vi "Rd Wr settings json Filter Wheel Table.vi"(8 "error in (no error)":errorcluster, 9 "Settings File":string="FilterWheelTable.json", 10 "Write? (F:Read)":bool, 11 "Filter Wheel Table":cluster{i32[], bool}[][](array[cluster])=[[{[], TRUE}, {[2800], TRUE}, {[2800, 2800], TRUE}, {[950, 1850], FALSE}], [{[2800], FALSE}, {[], TRUE}, {[2800], TRUE}, {[2800, 2800], TRUE}], [{[2800, 2800], FALSE}, {[2800], FALSE}, {[], TRUE}, {[2800], TRUE}], [{[2800, 2800], TRUE}, {[2800, 2800], FALSE}, {[2800], FALSE}, {[], TRUE}]]) -> (0 "error out":errorcluster, 3 "Filter Wheel Table":cluster{i32[], bool}[][](array[cluster])=[[{[], TRUE}, {[2800], TRUE}, {[2800, 2800], TRUE}, {[950, 1850], FALSE}], [{[2800], FALSE}, {[], TRUE}, {[2800], TRUE}, {[2800, 2800], TRUE}], [{[2800, 2800], FALSE}, {[2800], FALSE}, {[], TRUE}, {[2800], TRUE}], [{[2800, 2800], TRUE}, {[2800, 2800], FALSE}, {[2800], FALSE}, {[], TRUE}]])   [LabVIEW 2024]
uses:
  2e80df6d-94aa-46b9-8b94-ceea8c057880.vi
  659fb017-0e9f-42f9-b06e-930303f00cbc.vi
  <vilib>/JDP Science/JSONtext/Find Item.vi
  <vilib>/JDP Science/JSONtext/Next JSON Value.vi
  <vilib>/JDP Science/JSONtext/String Subset.vi
  <vilib>/JDP Science/JSONtext/Parsing/Advance past next JSON Value (inlined COPY).vi
  <vilib>/JDP Science/JSONtext/Parsing/Advance past whitespace.vi
  <vilib>/JDP Science/JSONtext/Parsing/Advance past String.vi
  <vilib>/JDP Science/JSONtext/Parsing/Advance past Number.vi
  <vilib>/JDP Science/JSONtext/Parsing/Advance past Line Ending.vi
  <vilib>/JDP Science/JSONtext/Parsing/Parse Full Path or Item Name.vi
  <vilib>/JDP Science/JSONtext/Parsing/Advance past Array.vi
  <vilib>/JDP Science/JSONtext/Parsing/Advance past Object.vi
  <vilib>/JDP Science/JSONtext/support/Error Cluster From Code.vi
  <vilib>/JDP Science/JSONtext/Offset/Find Item Locations by Path.vi
  <vilib>/JDP Science/JSONtext/JSON text to Variant.vi
  <vilib>/JDP Science/JSONtext/Variant to JSON Text.vi
  <vilib>/JDP Science/JSONtext/Set Item.vi
  <vilib>/JDP Science/JSONtext/LVClass Serializer/JSONtext LVClass Serializer.lvclass
  <vilib>/JDP Science/JSONtext/JSONtext.lvlib
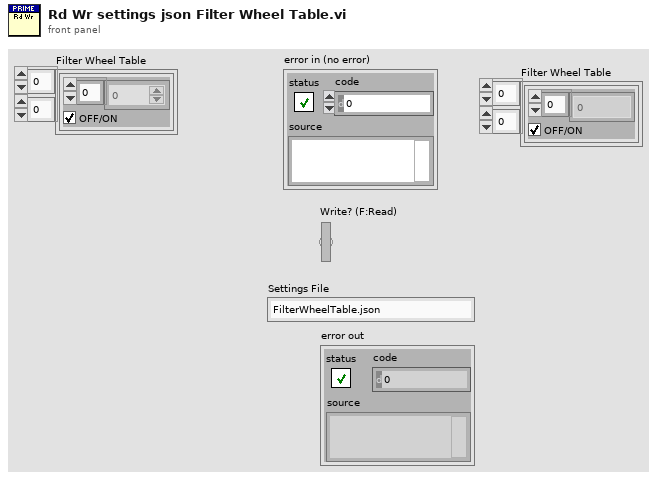
[diagram p1: front panel]
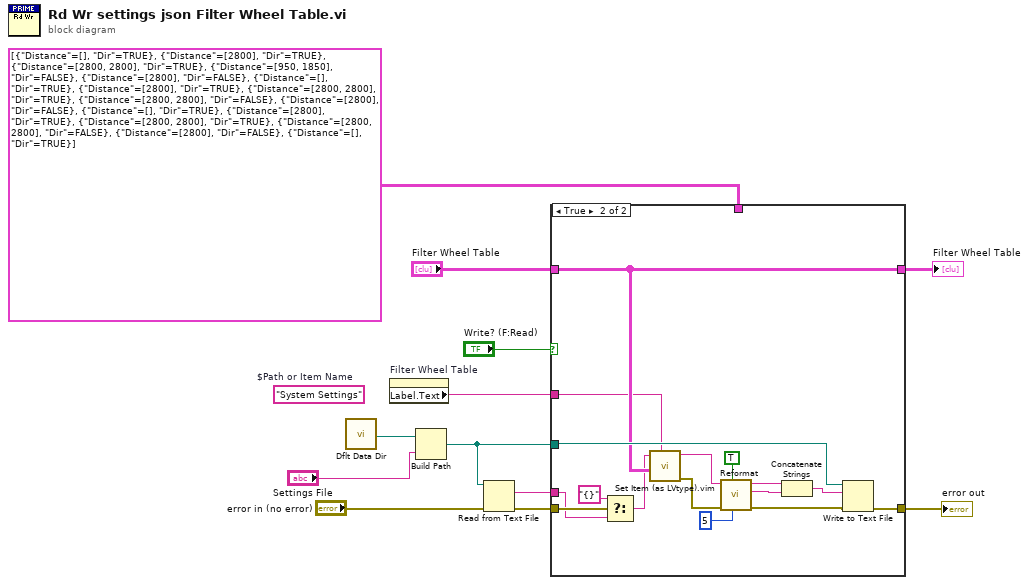
[diagram p0: block diagram]
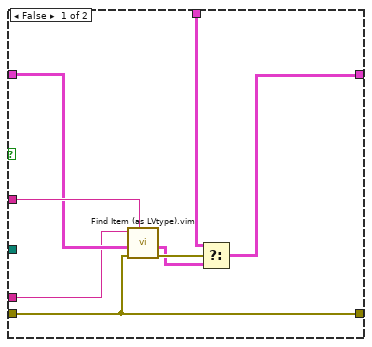
[diagram p2: hidden frame]
diagram:
  (unwired) "System Settings"  # $Path or Item Name
  n1 = call <vilib>:"Dflt Data Dir.vi"() -> ("App:Default Data Directory"=w9:path)
  n2 = property on="Filter Wheel Table" class="Arr (strict)"() -> ("Label.Text"=w2:string)  [unwired: 2 in, 2 out]
  n3 = Build Path(base path=w9, name or relative path="Settings File") -> (appended path=w3:path)
  n4 = Read from Text File(file (use dialog)=w3, error in="error in (no error)") -> (text=w4:string, error out=w5:errorcluster)  [unwired: 2 in, 2 out]
  n5 = case shown="True" "Write? (F:Read)" {
    tunnel: w5 -> [w14 w32]
    tunnel: "Filter Wheel Table" -> [w18 w34]
    tunnel: w3 -> [_ w36]
    tunnel: [w14 w35] -> w8
    tunnel: [w20 w34] -> w7
    tunnel: w2 -> [w19 w33]
    tunnel: w4 -> [w15 w30]
    tunnel: cluster{"Distance":i32[], "Dir":bool}[][] [[{"Distance"=[], "Dir"=TRUE}, {"Distance"=[2800], "Dir"=TRUE}, {"Distance"=[2800, 2800], "Dir"=TRUE}, {"Distance"=[950, 1850], "Dir"=FALSE}], [{"Distance"=[2800], "Dir"=FALSE}, {"Distance"=[], "Dir"=TRUE}, {"Distance"=[2800], "Dir"=TRUE}, {"Distance"=[2800, 2800], "Dir"=TRUE}], [{"Distance"=[2800, 2800], "Dir"=FALSE}, {"Distance"=[2800], "Dir"=FALSE}, {"Distance"=[], "Dir"=TRUE}, {"Distance"=[2800], "Dir"=TRUE}], [{"Distance"=[2800, 2800], "Dir"=TRUE}, {"Distance"=[2800, 2800], "Dir"=FALSE}, {"Distance"=[2800], "Dir"=FALSE}, {"Distance"=[], "Dir"=TRUE}]] -> [w13 _]
    frame False {
      n6 = call "Find Item (as LVtype).vim"("$Path or Item Name"=w19, "error in (no error)"=w14, "Data Type and Default Value"=w18, "JSON"=w15) -> ("error out"=w17:errorcluster, "Data"=w16:cluster{i32[], bool}[][])  [unwired: 4 in, 2 out]
      n7 = Select(t=w13, s=w17, f=w16) -> (s? t:f=w20:cluster{"Distance":i32[], "Dir":bool}[][])
    }
    frame True {
      n8 = Select(t="{}" ("JSON"), s=w32, f=w30) -> (s? t:f=w29:string)
      n9 = call "Set Item (as LVtype).vim"("$Path or Item Name"=w33, "Anything"=w34, "JSON"=w29) -> ("error out"=w22:errorcluster, "<JSON>"=w24:string)  [unwired: 5 in, 1 out]
      n10 = call <vilib>:"Reformat.vi"("Pretty Print Levels"=5, "Alphabetically Sort Objects"=TRUE, "error in (no error)"=w22, "JSON"=w24) -> ("error out"=w23:errorcluster, "Rest of Input String"=w28:string, "<JSON>"=w25:string)  [unwired: 4 in, 1 out]
      n11 = Concatenate Strings(w25, w28) -> (w21:string)
      n12 = Write to Text File(file (use dialog)=w36, text=w21, error in=w23) -> (error out=w35:errorcluster)  [unwired: 1 in, 2 out]
    }
  }
  "error out" <- w8
  "Filter Wheel Table" <- w7
